vi "Get Distance From AnchorDistanceArray By TagID.vi"(9 "Tag.lvclass":refnum<class "Tag.lvclass">, 10 "Input TagDistanceArray":T1(array[cluster])) -> (2 "Distance":dbl)   [LabVIEW 2014]
doc: "Purpose of this VI is to retrieve the specific\ndistance to a Tag from Anchor by extracting\nits value from the TagDistanceArray"
uses:
  Tag.lvclass
panel:
  out "error out":errorcluster
  in  "error in (no error)":errorcluster
  # "Purpose of this VI is to retrieve the specific\ndistance to a Tag from Anchor by extracting\nits value from the TagDistanceArray"
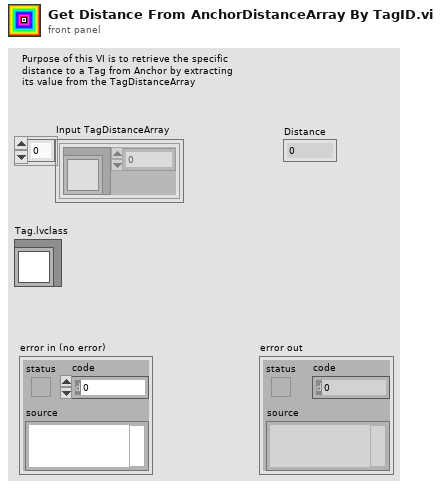
[diagram p1: front panel]
types:
  T1 = cluster{"Tag.lvclass":refnum<class "Tag.lvclass">, "Distance":dbl}[]
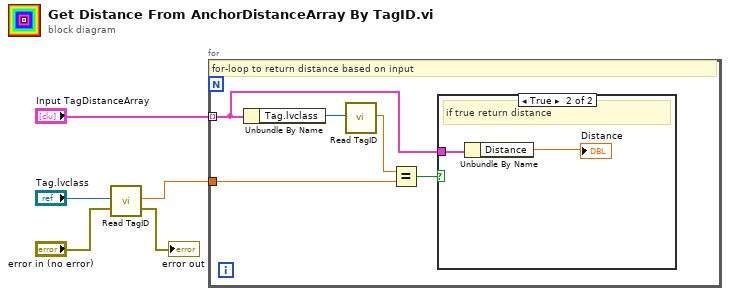
[diagram p0: block diagram]
diagram:
  n1 = call "Read TagID.vi"("Tag in"="Tag.lvclass", "error in (no error)"="error in (no error)") -> ("TagID"=w2:dbl, "error out"=→"error out":errorcluster)  [unwired: 15 in, 1 out]
  n2 = for {
    tunnel: "Input TagDistanceArray" -> [w8] mode=indexing
    tunnel: w2 -> [w10]
    # "for-loop to return distance based on input"
    n3 = Unbundle By Name(w8) -> ("Tag.lvclass"=w7:refnum<class "Tag.lvclass">)
    n4 = call "Read TagID.vi"("Tag in"=w7) -> ("TagID"=w6:dbl)  [unwired: 16 in, 2 out]
    n5 = Equal?(x=w6, y=w10) -> (x = y?=w9:bool)
    n6 = case shown="True" w9 {
      tunnel: w8 -> [_ w12]
      frame False {
        # "TODO what if false?\ncontinue loop\nwhat if loop end and nothing found?"
      }
      frame True {
        # "if true return distance"
        n7 = Unbundle By Name(w12) -> ("Distance"=→"Distance":dbl)
      }
    }
  }
